vi "Test-Reservation.vi"() -> ()   [LabVIEW 2013]
uses:
  src/SMO/Typedefs/Reserve State--Enum.ctl
  src/SMO.Example/SMO.Example.lvclass
  src/SMO/Typedefs/SMOState --Enum.ctl
  src/SMO/SMO.lvclass
panel:
  in  "Reserve":bool
  in  "Lock Key":string="myKey"
  out "Reserve State":T1
  in  "Unreserve Dependency":bool
  in  "Stop":bool
  out "error":errorcluster
  # "Reserve will set the key to \"myKey\".\n\nTo unreserve successfully, set Lock\nKey to \"myKey\". Any other key should\nfail to unreserve the resource.\n\nIn this example, the \"Check Availability\" method is\nconfigured to produce an error when denied access."
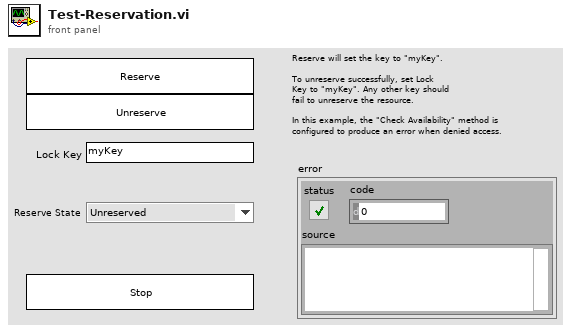
[diagram p1: front panel]
types:
  T1 = typedef "SMO.lvclass/Reserve State--Enum.ctl" = enum16{"Unreserved", "Reserved", "Self-locked"}
  T2 = typedef "SMO.lvclass/Public Events.ctl" = cluster{"Error":refnum<user-event>, "State":refnum<user-event>, "Reserve State":refnum<user-event>}
  T3 = cluster{"Event Registration Refnum":refnum<event-registration>, "Event Registration Refnum":refnum<event-registration>}
  T4 = typedef "SMO.lvclass/SMOState --Enum.ctl" = enum16{"unknown", "Created", "Started", "Stopped"}
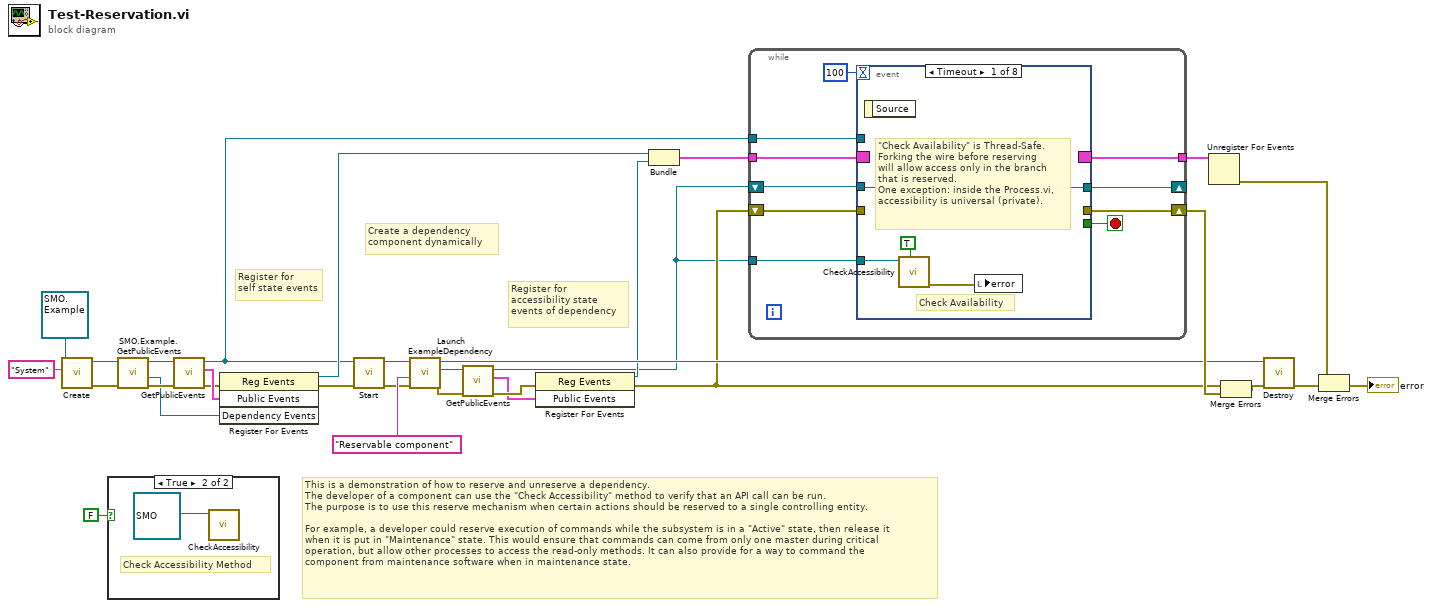
[diagram p0: block diagram]
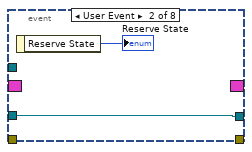
[diagram p3: hidden frame]
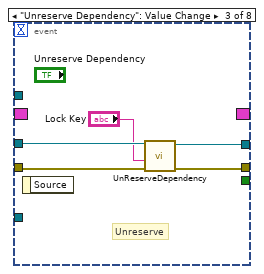
[diagram p4: hidden frame]
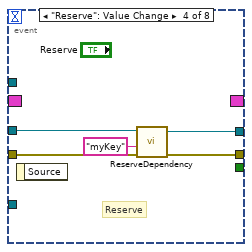
[diagram p5: hidden frame]
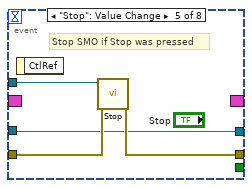
[diagram p6: hidden frame]
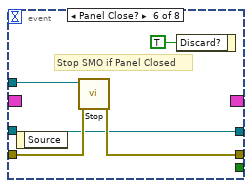
[diagram p7: hidden frame]
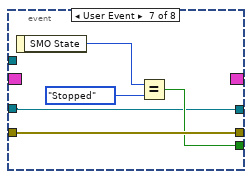
[diagram p8: hidden frame]
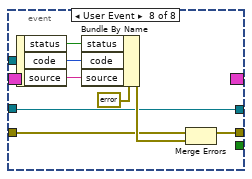
[diagram p9: hidden frame]
diagram:
  # "Create a dependency\ncomponent dynamically"
  # "Register for\nself state events"
  # "Register for\naccessibility state\nevents of dependency"
  # "This is a demonstration of how to reserve and unreserve a dependency.\nThe developer of a component can use the \"Check Accessibility\" method to verify that an API call can be run.\nThe purpose is to use this reserve mechanism when certain actions should be reserved to a single controlling entity.\n\nFor example, a developer could reserve execution of commands while the subsystem is in a \"Active\" state, then release it\nwhen it is put in \"Maintenance\" state. This would ensure that commands can come from only one master during critical\noperation, but allow other processes to access the read-only methods. It can also provide for a way to command the\ncomponent from maintenance software when in maintenance state."
  n1 = call "Create.vi"("Subsystem Name (optional)"="System", "SMO"=refnum<class "SMO.Example.lvclass"> refnum ("SMO.Example.lvclass")) -> ("error out"=w17:errorcluster, "SMO out"=w19:refnum<class "SMO.Example.lvclass">)  [unwired: 7 in, 1 out]
  n2 = case shown="True" FALSE {
    frame False {
    }
    frame True {
      # "Check Accessibility Method"
      n3 = call "CheckAccessibility.vi"("SMO in"=refnum<class "SMO.lvclass"> refnum ("SMO")) -> ()  [unwired: 8 in, 3 out]
    }
  }
  n4 = call "SMO.Example.GetPublicEvents.vi"("error in (no error)"=w17, "SMO.Example"=w19) -> ("error out"=w16:errorcluster, "Dependency Events"=w15:refnum<user-event>, "SMO.Example out"=w18:refnum<class "SMO.Example.lvclass">)  [unwired: 6 in, 1 out]
  n5 = call "GetPublicEvents.vi"("error in (no error)"=w16, "SMO"=w18) -> ("error out"=w23:errorcluster, "Public Events"=w24:T2, "SMO out"=w10:refnum<class "SMO.Example.lvclass">)  [unwired: 7 in]
  n6 = register-events(error in=w23, w24, w15) -> (reference out=w26:refnum<event-registration>, error out=w25:errorcluster)  [unwired: 1 in]
  n7 = call "Start.vi"("error in (no error)"=w25, "SMO"=w10) -> ("error out"=w11:errorcluster, "SMO out"=w14:refnum<class "SMO.Example.lvclass">)  [unwired: 8 in]
  n8 = call "Launch ExampleDependency.vi"("error in (no error)"=w11, "Name"="Reservable component" ("Subsystem Name (optional)"), "SMO.Example in"=w14) -> ("error out"=w6:errorcluster, "Dependency Reference"=w7:refnum<class "SMO.lvclass">, "SMO.Example out"=w12:refnum<class "SMO.Example.lvclass">)  [unwired: 5 in, 1 out]
  n9 = call "GetPublicEvents.vi"("error in (no error)"=w6, "SMO"=w7) -> ("error out"=w5:errorcluster, "Public Events"=w4:T2, "SMO out"=w2:refnum<class "SMO.lvclass">)  [unwired: 7 in]
  n10 = register-events(error in=w5, w4) -> (reference out=w3:refnum<event-registration>, error out=w8:errorcluster)  [unwired: 1 in]
  n11 = Bundle("Event Registration Refnum"=w26, "Event Registration Refnum"=w3) -> (w30:T3)  [unwired: 1 in]
  n12 = while {
    shift-right: [w37] -> w21
    shift-left: w8 -> [w41]
    tunnel: w30 -> [w40]
    tunnel: [w39] -> w31
    tunnel: w10 -> [w38]
    shift-right: [w35] -> _
    shift-left: w2 -> [w36]
    tunnel: w2 -> [w34]
    stop <- w42 stop-if-true
    n13 = event shown="[0] Timeout" {
      selector: w40 -> [_ _ _ _ _ _ _ _]
      dyn-events: [_ _ _ _ _ _ _ _] -> w39
      timeout: 100 -> [_ _ _ _ _ _ _ _]
      tunnel: [_ _ _ _ _ _ w69 _] -> w42
      tunnel: w38 -> [_ _ _ _ w62 w67 _ _]
      tunnel: [_ _ w51 w56 w61 w66 w70 w74] -> w37
      tunnel: w41 -> [_ _ w52 w57 w60 w65 w70 w75]
      tunnel: w36 -> [w46 w47 w53 w58 w59 w63 w68 w73]
      tunnel: [w46 w47 w49 w54 w59 w63 w68 w73] -> w35
      tunnel: w34 -> [w45 _ _ _ _ _ _ _]
      event Timeout {
        # "\"Check Availability\" is Thread-Safe.\nForking the wire before reserving\nwill allow access only in the branch\nthat is reserved.\nOne exception: inside the Process.vi,\naccessibility is universal (private)."
        # "Check Availability"
        n14 = event-data() -> ()  [unwired: 1 in, 1 out]
        n15 = call "CheckAccessibility.vi"("Error if denied? (F)"=TRUE, "SMO in"=w45) -> ("error out"=w44:errorcluster)  [unwired: 7 in, 2 out]
        n16 = local write "error"(w44) -> ()
      }
      event User Event {
        n17 = event-data() -> ("Reserve State"=→"Reserve State":T1)  [unwired: 1 in]
      }
      event "Unreserve Dependency": Value Change {
        # "Unreserve"
        n18 = event-data() -> ()  [unwired: 1 in, 1 out]
        n19 = call "UnReserveDependency.vi"("error in (no error)"=w52, "Lock Key (if no reserving entity)"="Lock Key", "SMO"=w53) -> ("error out"=w51:errorcluster, "SMO out"=w49:refnum<class "SMO.lvclass">)  [unwired: 6 in, 1 out]
      }
      event "Reserve": Value Change {
        # "Reserve"
        n20 = event-data() -> ()  [unwired: 1 in, 1 out]
        n21 = call "ReserveDependency.vi"("error in (no error)"=w57, "Lock Key (if no reserving entity)"="myKey" ("Lock Key (if no controlling entity)"), "SMO"=w58) -> ("error out"=w56:errorcluster, "SMO out"=w54:refnum<class "SMO.lvclass">)  [unwired: 6 in, 1 out]
      }
      event "Stop": Value Change {
        # "Stop SMO if Stop was pressed"
        n22 = event-data() -> ()  [unwired: 1 in, 1 out]
        n23 = call "Stop.vi"("error in (no error)"=w60, "SMO"=w62) -> ("error out"=w61:errorcluster)  [unwired: 8 in, 1 out]
      }
      event Panel Close? {
        # "Stop SMO if Panel Closed"
        n24 = event-data() -> ()  [unwired: 1 in, 1 out]
        n25 = call "Stop.vi"("error in (no error)"=w65, "SMO"=w67) -> ("error out"=w66:errorcluster)  [unwired: 8 in, 1 out]
        n26 = event-data("Discard?"=TRUE ("OK")) -> ()  [unwired: 1 in, 1 out]
      }
      event User Event {
        n27 = event-data() -> ("SMO State"=w72:T4)  [unwired: 1 in]
        n28 = Equal?(x=w72, y=SMOState_--Enum."Stopped") -> (x = y?=w69:bool)
      }
      event User Event {
        n29 = event-data() -> ("status"=w80:bool, "code"=w78:i32, "source"=w77:string)  [unwired: 1 in]
        n30 = Bundle By Name(cluster=errorcluster {"status"=FALSE, "code"=0, "source"=""} ("error constant"), "status"=w80, "code"=w78, "source"=w77) -> (w76:errorcluster)
        n31 = Merge Errors(w75, w76) -> (w74:errorcluster)
      }
    }
  }
  n32 = Unregister For Events(event registration refnum=w31) -> (error out=w29:errorcluster)  [unwired: 1 in]
  n33 = Merge Errors(w8, w21) -> (w9:errorcluster)
  n34 = call "Destroy.vi"("error in (no error)"=w9, "SMO"=w12) -> ("error out"=w27:errorcluster)  [unwired: 9 in]
  n35 = Merge Errors(w29, w27) -> (→"error":errorcluster)
